vi "Polish Return Wire.vi"(10 "Return Wire":refnum<vi>, 11 "Abstract Param Writer in":refnum<class "Abstract Param Writer.lvclass">) -> (3 "Abstract Param Writer out":refnum<class "Abstract Param Writer.lvclass">)   [LabVIEW 2013, in "Abstract Param Writer.lvclass"]
doc: "Subclasses can reimplement this VI to manipulate the wire from the CLFN terminal to the indicator terminal (for example, to insert nodes along the path).\n\nThe default implementation leaves the wire in place and removes the template label."
uses:
  Abstract Param Writer.lvclass
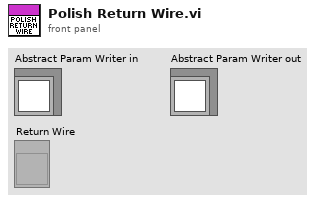
[diagram p1: front panel]
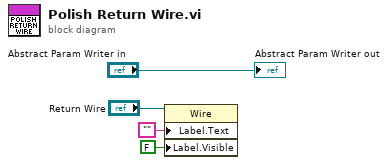
[diagram p0: block diagram]
diagram:
  n1 = property class="Wire"(reference="Return Wire", "Label.Text"="", "Label.Visible"=FALSE) -> ()  [unwired: 1 in, 2 out]
  "Abstract Param Writer out" <- "Abstract Param Writer in"
